vi "LakeShore218_read.vi"(8 "error in":errorcluster, 11 "VISA in":refnum<visa-resource-name>) -> (0 "error out":errorcluster, 2 "value_array":dbl[](array[numeric]), 3 "VISA out":refnum<visa-resource-name>, 4 "status":bool)   [LabVIEW 2019]
panel:
  out "string":string
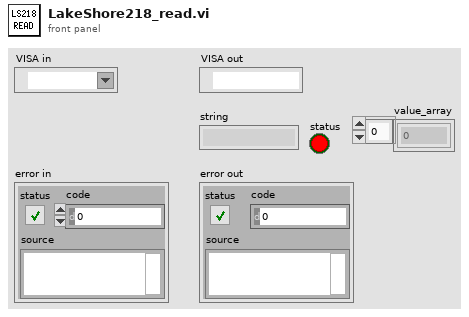
[diagram p1: front panel]
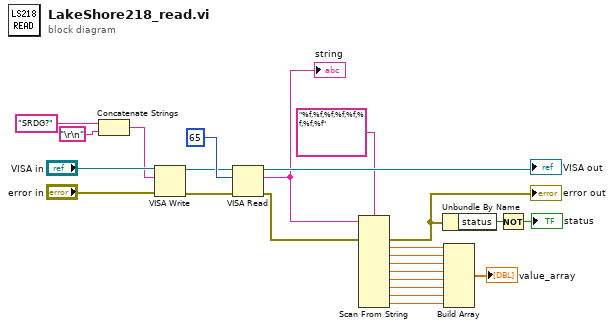
[diagram p0: block diagram]
diagram:
  n1 = Concatenate Strings("SRDG?" ("write buffer 2"), "\r\n") -> (w19:string)
  n2 = VISA Write(VISA resource name="VISA in", write buffer=w19, error in (no error)="error in") -> (VISA resource name out=w21:refnum<visa-resource-name>, error out=w22:errorcluster)  [unwired: 1 out]
  n3 = VISA Read(VISA resource name=w21, byte count=u32 65, error in (no error)=w22) -> (VISA resource name out=→"VISA out":refnum<visa-resource-name>, read buffer=w15:string, error out=w13:errorcluster)  [unwired: 1 out]
  "string" <- w15
  n4 = Scan From String(format string="%f,%f,%f,%f,%f,%f,%f,%f", input string=w15, error in=w13) -> (error out=w12:errorcluster, output 1=w9:dbl, output 2=w8:dbl, output 3=w7:dbl, output 4=w6:dbl, output 5=w5:dbl, output 6=w4:dbl, output 7=w3:dbl, output 8=w2:dbl)  [unwired: 9 in, 2 out]
  "error out" <- w12
  n5 = Unbundle By Name(w12) -> ("status"=w11:bool)
  n6 = Build Array(w9, w8, w7, w6, w5, w4, w3, w2) -> (→"value_array":dbl[])
  n7 = Not(x=w11) -> (.not. x?=→"status":bool)
